vi "Pathfind.vi"(0 "Start Vector":cluster{"x":dbl, "y":dbl, "angle":dbl}, 1 "Destination":cluster{"x":dbl, "y":dbl, "angle":dbl}, 2 "Pathfinding Settings":T1={"Movement Settings"={"Arrival Tolerance (m)"=0.01, "Closeness Threshold (m)"=0.5, "Pit Obstacle Radius (m)"=0.5, "Pit Locations"=[]}, "Dead Zone"=0.75, "Max Moves"=3.0, "Move Segment Length (m)"=0.02, "Path Cost Weights"={"Length Weight"=1.0, "Angle Weight"=0.0, "Angle Error Weight"=1000.0, "Angle Error Threshold"=0.314, "Per Move Penalty"=0.05, "Closeness Weight"=100.0, "Too Short Penalty"=100.0, "Too Short Threshold"=1.5}, "Desperation - Reduction Per Attempt (Ratio)"=0.9, "Desperation - Max Attempts"=1, "Log All Move Points"=FALSE, "Intermediate Position Grids"=[{"x1"=0.0, "x2"=1.75, "resolution"=0.15}, {"x1"=1.75, "x2"=7.38, "resolution"=0.4}]}, 3 "Specified End Angle":bool, 4 "Turn Radius (m)":dbl) -> (5 "Best Path":T5, 6 "Used Turn Radius (m)":dbl, 7 "Total Paths Arrived":dbl, 8 "Total Paths Checked":dbl)   [LabVIEW 2015, in "Navigation2017.lvlib"]
uses:
  Navigation2017.lvlib
  Path.ctl
  Move.ctl
  PathfindingSettings.ctl
  MovementSettings.ctl
  PathCostWeights.ctl
  IntermediatePositionGrids.ctl
  Navigation2017-SubVIs.lvlib
panel:
  # "OUTPUTS"
  # "INPUTS"
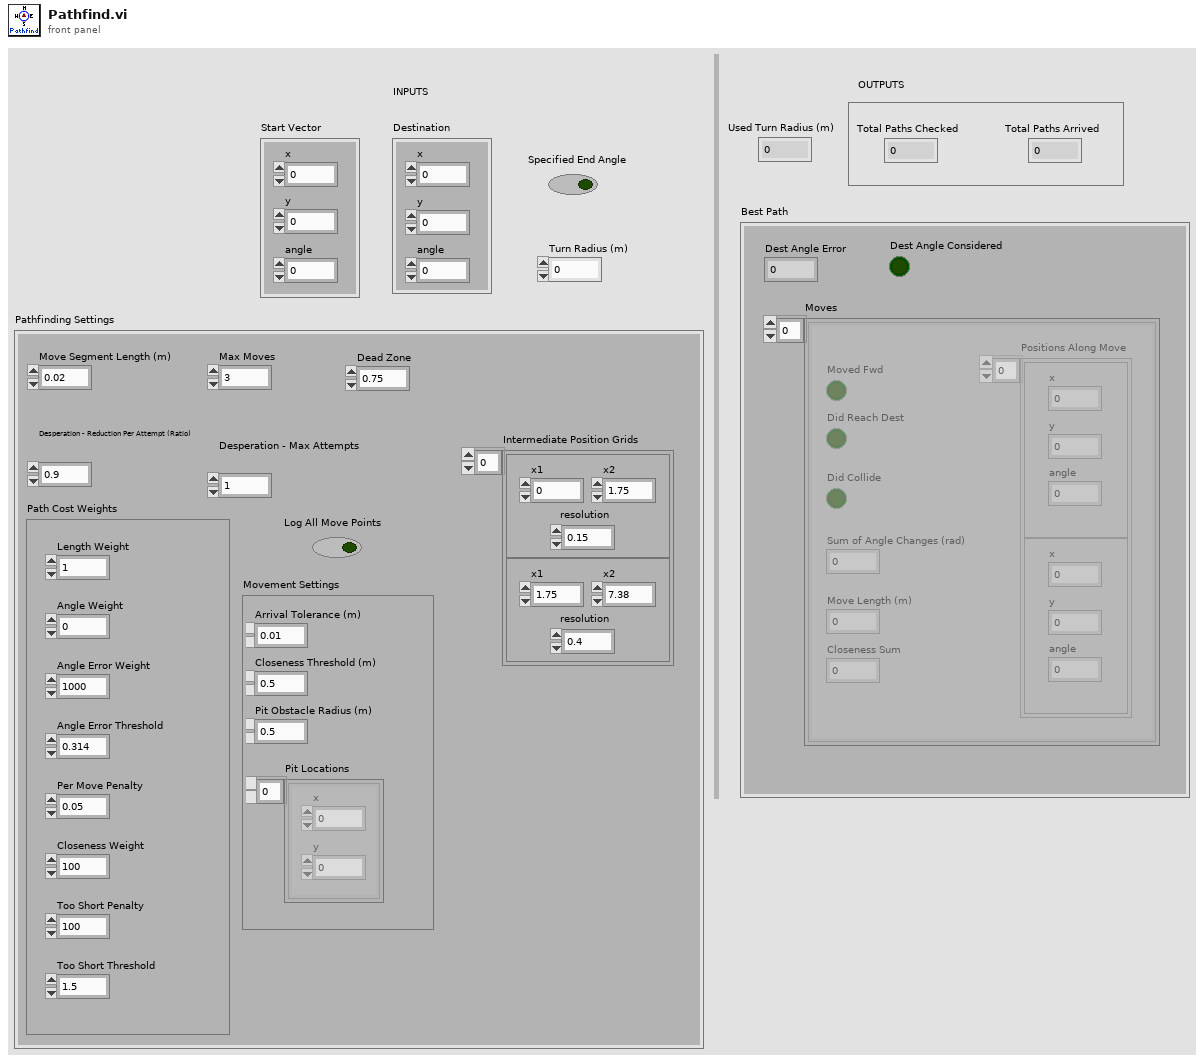
[diagram p1: front panel]
types:
  T1 = typedef "Navigation2017.lvlib/PathfindingSettings.ctl" = cluster{"Movement Settings":T2, "Dead Zone":dbl, "Max Moves":dbl, "Move Segment Length (m)":dbl, "Path Cost Weights":T3, "Desperation - Reduction Per Attempt (Ratio)":dbl, "Desperation - Max Attempts":i16, "Log All Move Points":bool, "Intermediate Position Grids":T4}
  T2 = typedef "Navigation2017.lvlib/MovementSettings.ctl" = cluster{"Arrival Tolerance (m)":dbl, "Closeness Threshold (m)":dbl, "Pit Obstacle Radius (m)":dbl, "Pit Locations":cluster{"x":dbl, "y":dbl}[]}
  T3 = typedef "Navigation2017.lvlib/PathCostWeights.ctl" = cluster{"Length Weight":dbl, "Angle Weight":dbl, "Angle Error Weight":dbl, "Angle Error Threshold":dbl, "Per Move Penalty":dbl, "Closeness Weight":dbl, "Too Short Penalty":dbl, "Too Short Threshold":dbl}
  T4 = typedef "Navigation2017.lvlib/IntermediatePositionGrids.ctl" = cluster{"x1":dbl, "x2":dbl, "resolution":dbl}[]
  T5 = typedef "Navigation2017.lvlib/Path.ctl" = cluster{"Dest Angle Error":dbl, "Dest Angle Considered":bool, "Moves":T6[]}
  T6 = typedef "Navigation2017.lvlib/Move.ctl" = cluster{"Did Reach Dest":bool, "Did Collide":bool, "Sum of Angle Changes (rad)":dbl, "Move Length (m)":dbl, "Closeness Sum":dbl, "Positions Along Move":cluster{"x":dbl, "y":dbl, "angle":dbl}[], "Moved Fwd":bool}
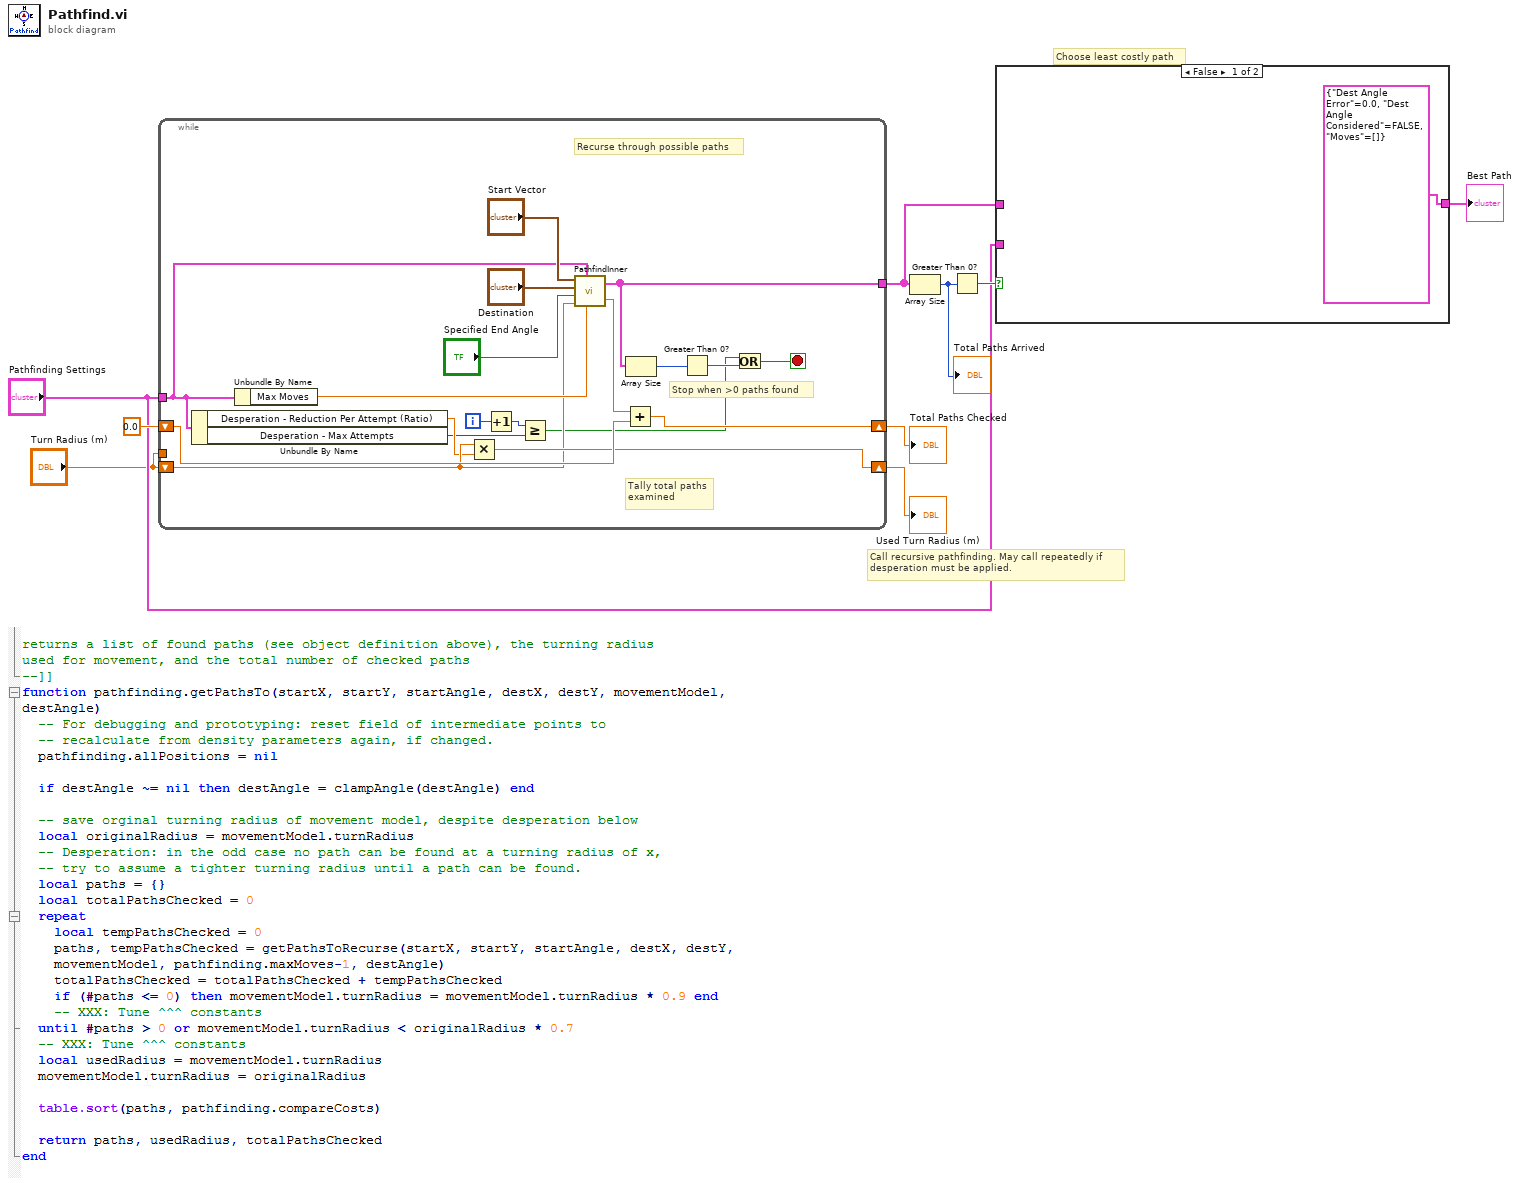
[diagram p0: block diagram]
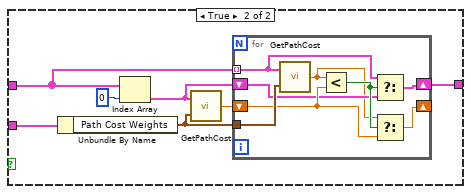
[diagram p2: hidden frame]
diagram:
  # "Choose least costly path"
  # "Call recursive pathfinding. May call repeatedly if\ndesperation must be applied."
  n1 = while {
    shift-right: [w22] -> w7
    shift-left: 0.0 -> [w23]
    shift-right: [w18] -> w8
    shift-left: "Turn Radius (m)" -> [w17]
    tunnel: [w16] -> w4
    tunnel: "Pathfinding Settings" -> [w14]
    tunnel: "Turn Radius (m)" -> [_]
    i -> [w10]
    stop <- w19 stop-if-true
    # "Stop when >0 paths found"
    # "Tally total paths\nexamined"
    # "Recurse through possible paths"
    n2 = Unbundle By Name(w14) -> ("Desperation - Reduction Per Attempt (Ratio)"=w15:dbl, "Desperation - Max Attempts"=w12:i16)
    n3 = Unbundle By Name(w14) -> ("Max Moves"=w25:dbl)
    n4 = Multiply(x=w17, y=w15) -> (x*y=w18:dbl)
    n5 = Increment(x=w10) -> (x+1=w11:i32)
    n6 = Greater Or Equal?(x=w11, y=w12) -> (x >= y?=w13:bool)
    n7 = call "PathfindInner.vi"("Moves Left"=w25, "Pathfinding Settings"=w14, "Turn Radius (m)"=w17, "Specified End Angle"="Specified End Angle", "Destination"="Destination", "Start Vector"="Start Vector") -> ("Total Paths Checked"=w24:dbl, "Paths To Dest"=w16:T5[])
    n8 = Add(x=w24, y=w23) -> (x+y=w22:dbl)
    n9 = Array Size(array=w16) -> (size(s)=w21:i32)
    n10 = Greater Than 0?(x=w21) -> (x > 0?=w20:bool)
    n11 = Or(x=w13, y=w20) -> (x .or. y?=w19:bool)
  }
  "Used Turn Radius (m)" <- w8
  "Total Paths Checked" <- w7
  n12 = Array Size(array=w4) -> (size(s)=w5:i32)
  "Total Paths Arrived" <- w5
  n13 = Greater Than 0?(x=w5) -> (x > 0?=w6:bool)
  n14 = case shown="False" w6 {
    tunnel: w4 -> [_ w35]
    tunnel: "Pathfinding Settings" -> [_ w34]
    tunnel: [T5 {"Dest Angle Error"=0.0, "Dest Angle Considered"=FALSE, "Moves"=[]} ("Best Path") w30] -> w2
    frame False {
    }
    frame True {
      n15 = Unbundle By Name(w34) -> ("Path Cost Weights"=w33:T3)
      n16 = Index Array(array=w35, index=0) -> (element=w32:T5)
      n17 = call "GetPathCost.vi"("Path Cost Weights"=w33, "Path"=w32) -> ("Cost"=w31:dbl)
      n18 = for {
        shift-right: [w39] -> w30
        shift-left: w32 -> [w38]
        tunnel: w35 -> [w40] mode=indexing
        shift-right: [w41] -> _
        shift-left: w31 -> [w42]
        tunnel: w33 -> [w44]
        n19 = call "GetPathCost.vi"("Path Cost Weights"=w44, "Path"=w40) -> ("Cost"=w37:dbl)
        n20 = Less?(x=w37, y=w42) -> (x < y?=w43:bool)
        n21 = Select(t=w40, s=w43, f=w38) -> (s? t:f=w39:T5)
        n22 = Select(t=w37, s=w43, f=w42) -> (s? t:f=w41:dbl)
      }
    }
  }
  "Best Path" <- w2
